vi "targetsToString.vi"(9 "Column3":dbl[](array[numeric]), 10 "Column2":dbl[](array[numeric]), 11 "Column1":dbl[](array[numeric])) -> (3 "plotString":string)   [LabVIEW 2021]
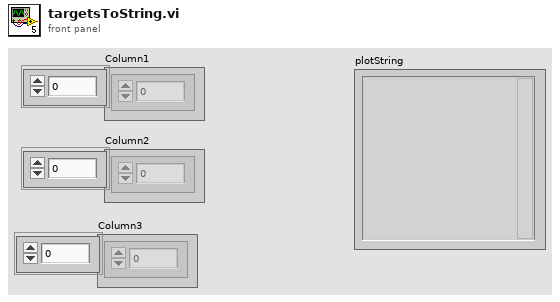
[diagram p1: front panel]
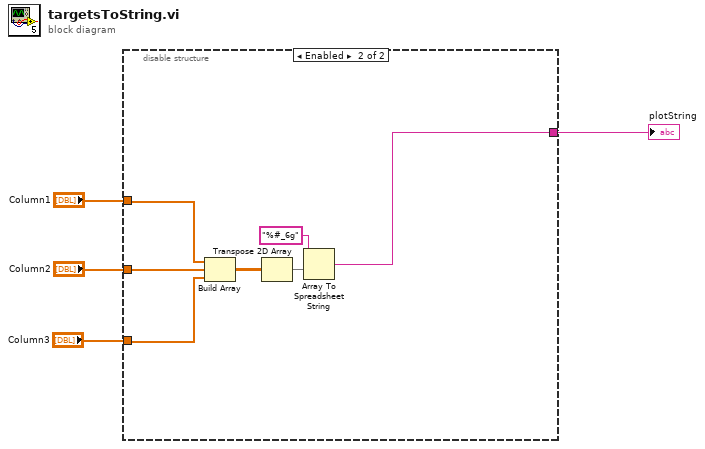
[diagram p0: block diagram]
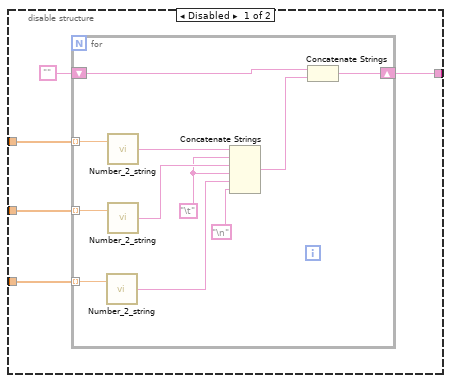
[diagram p2: hidden frame]
diagram:
  n1 = disable-structure shown="Enabled" {
    disable-tunnel: "Column1" -> [w7 w23]
    disable-tunnel: "Column2" -> [w6 w24]
    disable-tunnel: "Column3" -> [w5 w22]
    disable-tunnel: [w8 w21] -> w1
    frame Disabled {
      n2 = for {
        tunnel: w7 -> [w13] mode=indexing
        shift-right: [w17] -> w8
        shift-left: "" -> [w18]
        tunnel: w6 -> [w12] mode=indexing
        tunnel: w5 -> [w11] mode=indexing
        w15 = "\t"
        n3 = call "Number_2_string.vi"("number"=w11) -> ("String"=w10:string)  [unwired: 1 in]
        n4 = call "Number_2_string.vi"("number"=w13) -> ("String"=w20:string)  [unwired: 1 in]
        n5 = call "Number_2_string.vi"("number"=w12) -> ("String"=w19:string)  [unwired: 1 in]
        n6 = Concatenate Strings(w20, w15, w19, w15, w10, "\n") -> (w16:string)
        n7 = Concatenate Strings(w18, w16) -> (w17:string)
      }
    }
    frame Enabled {
      n8 = Build Array(w23, w24, w22) -> (w26:dbl[][])
      n9 = Transpose 2D Array(2D array=w26) -> (transposed array=w27:dbl[][])
      n10 = Array To Spreadsheet String(array=w27, 3:"%#_6g" ("format string")) -> (spreadsheet string=w21:string)  [unwired: 1 in]
    }
  }
  "plotString" <- w1
